vi "Min.vi"(10 "Value 2":u64, 11 "Value 1":u64) -> (2 "Value2 Smaller":bool, 3 "Min value":u64)   [LabVIEW 2023, in "2024_16.lvclass"]
uses:
  2024_16.lvclass
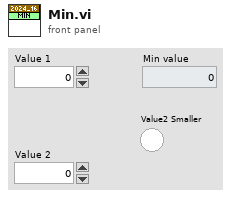
[diagram p1: front panel]
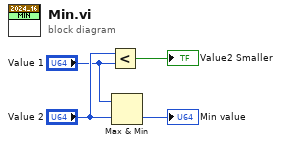
[diagram p0: block diagram]
diagram:
  n1 = Less?(x="Value 2", y="Value 1") -> (x < y?=→"Value2 Smaller":bool)
  n2 = Max & Min(x="Value 1", y="Value 2") -> (min(x,y)=→"Min value":u64)  [unwired: 1 out]
